vi "CreateDataEvent.vi"(7 "Qbus":refnum<class "Qbus.lvclass">, 8 "error in (no error)":errorcluster, 9 "data flow":T5, 10 "data event config":T2, 11 "config":T1) -> (0 "error out":errorcluster, 3 "config out":T1)   [LabVIEW 2017, in "EmsaDataEventCreator.lvlib"]
uses:
  <vilib>/addons/InsightCM/Devices/Shared/Emsa/EmsaDataEventCreator/EmsaDataEventCreator.lvlib
  <vilib>/addons/Qbus/Qbus.lvclass
  <vilib>/addons/InsightCM/Devices/Shared/Common/DataFlow/controls/Data.ctl
  <vilib>/addons/InsightCM/Utilities/DataAccessors/controls/wfmSGL_DVR.ctl
  <vilib>/addons/PointValueMap/controls/PointMap.ctl
  <vilib>/addons/InsightCM/Devices/Shared/Common/DataFlow/controls/Type.ctl
  <vilib>/addons/InsightCM/Devices/Shared/Emsa/EmsaDataEventCreator/controls/DataEventConfig.ctl
  <vilib>/addons/InsightCM/Devices/Shared/Emsa/EmsaDataEventCreator/controls/SweepParams.ctl
  <vilib>/addons/InsightCM/Devices/Shared/Emsa/EmsaDataEventCreator/controls/config.ctl
  <vilib>/addons/InsightCM/Devices/Shared/Common/FileFlow/subVIs/GetFirstProcessModule_EventRef.vi
  <vilib>/addons/InsightCM/Devices/Shared/Common/FileFlow/FileFlow.lvlib
  <vilib>/addons/InsightCM/Devices/Shared/Common/DataEventCreator/DataEventCreator.lvlib
  <vilib>/addons/PointValueMap/PointValueMap.lvlib
  <vilib>/addons/InsightCM/Devices/Shared/Common/DataFlow/DataFlow.lvlib
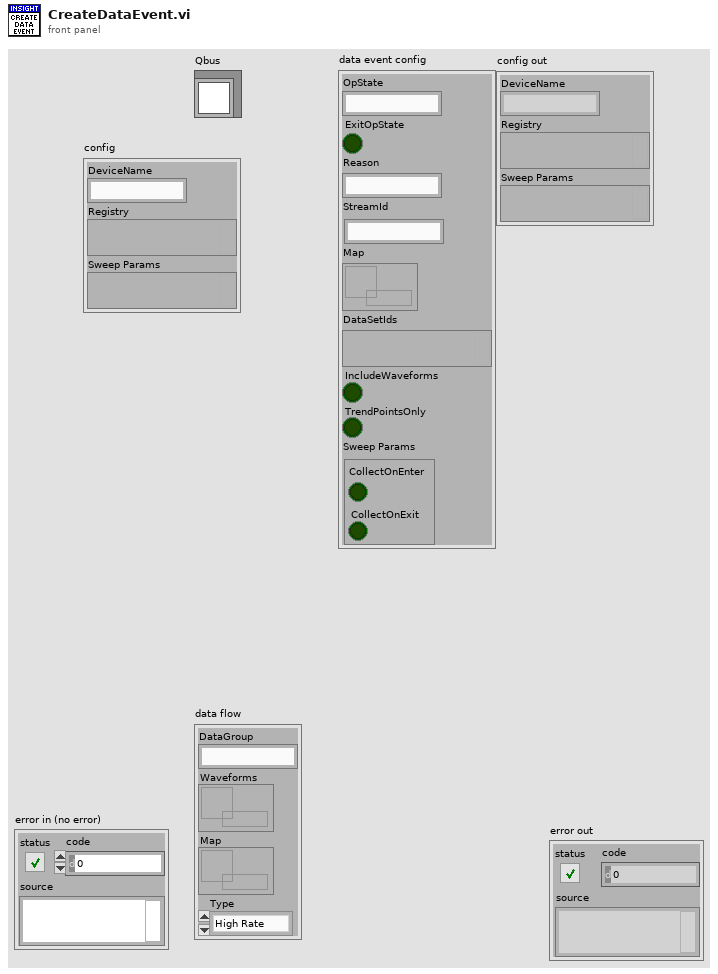
[diagram p1: front panel]
types:
  T1 = typedef "EmsaDataEventCreator.lvlib/config.ctl" = cluster{"DeviceName":string, "Registry":variant, "Sweep Params":variant}
  T2 = typedef "EmsaDataEventCreator.lvlib/DataEventConfig.ctl" = cluster{"OpState":string, "ExitOpState":bool, "Reason":string, "StreamId":string, "Map":T3, "DataSetIds":variant, "IncludeWaveforms":bool, "TrendPointsOnly":bool, "Sweep Params":T4}
  T3 = typedef "PointValueMap.lvlib/PointMap.ctl" = refnum<data-value>
  T4 = typedef "EmsaDataEventCreator.lvlib/SweepParams.ctl" = cluster{"CollectOnEnter":bool, "CollectOnExit":bool}
  T5 = typedef "DataFlow.lvlib/Data.ctl" = cluster{"DataGroup":string, "Waveforms":T6, "Map":T3, "Type":T7}
  T6 = typedef "wfmSGL_DVR.ctl" = refnum<data-value>
  T7 = typedef "DataFlow.lvlib/Type.ctl" = enum16{"High Rate", "Low Rate", "Burst Mode"}
  T8 = typedef "DataEvent.lvlib/Event.ctl" = cluster{"DataEvent":T9, "DataSets":T11[], "TrendPoints":T13[], "Alarms":T14[]}
  T9 = typedef "DataEvent.ctl" = cluster{"Id":string, "AssetNodeId":string, "Timestamp":i64, "Props":T10[]}
  T10 = typedef "KeyValuePair.ctl" = cluster{"Key":string, "Value":string}
  T11 = typedef "DataEvent.lvlib/DataSet.ctl" = cluster{"DataSetMetadata":T12, "Values":sgl[], "Values DVR":refnum<data-value>}
  T12 = typedef "DataSetMetadata.ctl" = cluster{"Id":string, "DataEventId":string, "AssetNodeId":string, "Type":string, "T0":i64, "Props":T10[]}
  T13 = typedef "TrendPoint.ctl" = cluster{"TrendPointId":string, "DataEventId":string, "Timestamp":i64, "Value":dbl, "Props":T10[]}
  T14 = typedef "TrendAlarmUpdate.ctl" = cluster{"RuleId":string, "Transition":T15}
  T15 = typedef "TrendAlarmTransition.ctl" = cluster{"At":i64, "Severity":i32, "Value":dbl, "Properties":T10[]}
  T16 = typedef "EmsaDataEventCreator.lvlib/Registry.ctl" = cluster{"Sweep Registry":T17[], "Trend Points":T19[], "AssetNodeMap":variant}
  T17 = typedef "EmsaDataEventCreator.lvlib/Registry_Sweep.ctl" = cluster{"Name":string, "DataSetType":T18, "Properties":T10[]}
  T18 = typedef "DataEvent.lvlib/DataSetType.ctl" = enum16{"Waveform", "SpeedProfile", "ThermalImage", "EmsaSweep"}
  T19 = typedef "DataEventCreator.lvlib/Registry_Trend.ctl" = cluster{"TrendPointId":string, "DataSetName":string, "HighRate":bool, "Always Send":bool}
  T20 = typedef "FileFlow.lvlib/data_eventRef.ctl" = cluster{"event reference":T21, "DataGroup":string, "OperatingState":string, "StreamId":string, "LastBlock":bool, "Map":T3, "TrendPoints Only":bool, "Extra Large File":bool}
  T21 = typedef "DataEvent.lvlib/EventReference.ctl" = refnum<data-value>
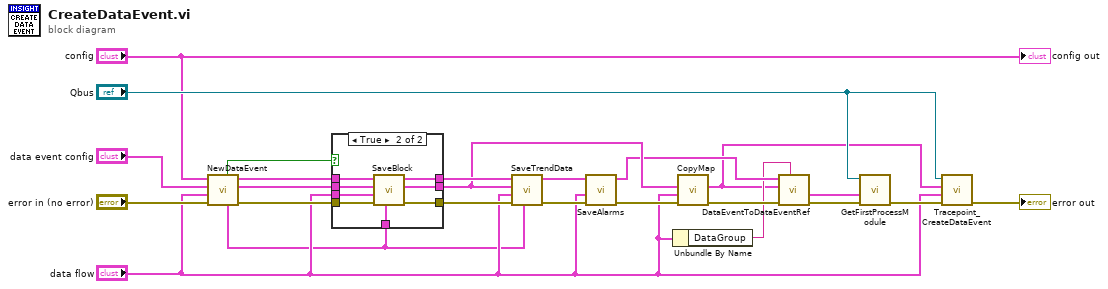
[diagram p0: block diagram]
diagram:
  n1 = call <vilib>:"NewDataEvent.vi"("error in (no error)"="error in (no error)", "data flow"="data flow", "data event config"="data event config", "config"="config") -> ("error out"=w16:errorcluster, "data event config"=w17:T2, "data event"=w11:T8, "registry"=w1:T16, "save waveforms"=w10:bool)  [unwired: 3 in]
  n2 = case shown="True" w10 {
    tunnel: [w27 w35] -> w19
    tunnel: [w25 w29] -> w18
    tunnel: w17 -> [w26 w34]
    tunnel: w16 -> [w27 w33]
    tunnel: "data flow" -> [_ w32]
    tunnel: w1 -> [_ w31]
    tunnel: w11 -> [w25 w30]
    tunnel: [w26 w28] -> w8
    frame False {
    }
    frame True {
      n3 = call <vilib>:"SaveBlock.vi"("registry"=w31, "error in (no error)"=w33, "data flow"=w32, "data event config"=w34, "data event"=w30) -> ("error out"=w35:errorcluster, "data event config out"=w28:T2, "data event out"=w29:T8)  [unwired: 4 in]
    }
  }
  n4 = call <vilib>:"SaveTrendData.vi"("registry"=w1, "error in (no error)"=w19, "data"="data flow", "data event config"=w8, "data event"=w18) -> ("error out"=w20:errorcluster, "data event out"=w9:T8)  [unwired: 5 in]
  n5 = call <vilib>:"SaveAlarms.vi"("error in (no error)"=w20, "data flow"="data flow", "data event"=w9) -> ("error out"=w7:errorcluster, "data event out"=w5:T8)  [unwired: 7 in]
  n6 = Unbundle By Name("data flow") -> ("DataGroup"=w4:string)
  n7 = call <vilib>:"CopyMap.vi"("error in (no error)"=w7, "data flow"="data flow", "data event config"=w8) -> ("error out"=w6:errorcluster, "data event config out"=w2:T2)  [unwired: 7 in]
  n8 = call <vilib>:"DataEventToDataEventRef.vi"("data group"=w4, "error in (no error)"=w6, "data event config"=w2, "data event"=w5) -> ("error out"=w13:errorcluster, "data event ref"=w14:T20)  [unwired: 6 in]
  n9 = call-poly <vilib>:"GetFirstProcessModule.vi"("error in (no error)"=w13, "data"=w14, "Qbus in"="Qbus") -> ("error out"=w15:errorcluster)  [unwired: 7 in, 1 out]
  n10 = call <vilib>:"Tracepoint_CreateDataEvent.vi"("error in (no error)"=w15, "data"="data flow", "data event config"=w2, "Qbus"="Qbus") -> ("error out"=→"error out":errorcluster)  [unwired: 7 in]
  "config out" <- "config"
